vi "Setup subWorkers.vi"(8 "error in":errorcluster, 11 "Maestro Control in":refnum<class "Maestro Control.lvclass">) -> (0 "error out":errorcluster, 3 "Maestro Control out":refnum<class "Maestro Control.lvclass">)   [LabVIEW 2021, in "Maestro Control.lvclass"]
doc: "<b>Note: Do not change the code in this VI!</b>\nThis VI performs a setup of all the statically-linked subWorkers that belong to the Worker that calls this VI. This VI is created automatically by the 'Create/Add Worker' tool and must be called <b>before</b> any statically linked subWorkers are called."
uses:
  Maestro Control.lvclass
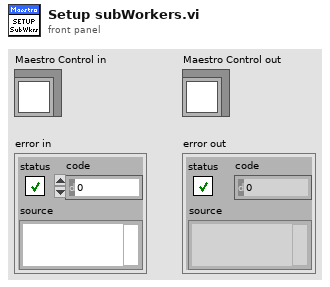
[diagram p1: front panel]
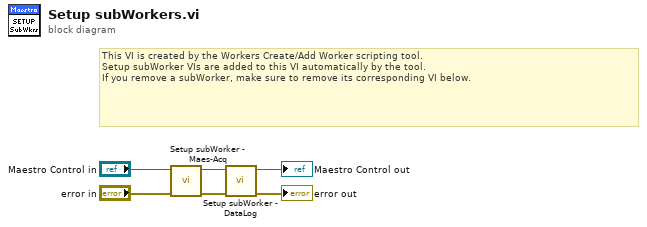
[diagram p0: block diagram]
diagram:
  # "This VI is created by the Workers Create/Add Worker scripting tool.\nSetup subWorker VIs are added to this VI automatically by the tool.\nIf you remove a subWorker, make sure to remove its corresponding VI below."
  n1 = call "Setup subWorker - Maes-Acq.vi"("error in"="error in", "Maestro Control in"="Maestro Control in") -> ("error out"=w5:errorcluster, "Maestro Control out"=w2:refnum<class "Maestro Control.lvclass">)  [unwired: 8 in]
  n2 = call "Setup subWorker - DataLog.vi"("error in"=w5, "Maestro Control in"=w2) -> ("error out"=→"error out":errorcluster, "Maestro Control out"=→"Maestro Control out":refnum<class "Maestro Control.lvclass">)  [unwired: 8 in]
